vi "DigInputs Write.vi"(4 "error in (no error)":errorcluster, 5 "Value":string[](array[string]), 6 "Container State":T2, 7 "Display State In":T1) -> (0 "error out":errorcluster, 3 "Display State Out":T1)   [LabVIEW 2015, in "Input Criteria Table.xctl"]
uses:
  Input Criteria Table.xctl
  <vilib>/_xctls/Container State.ctl
  State.vi
  <vilib>/_xctls/XControlSupport.lvlib
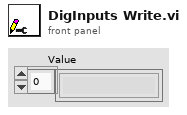
[diagram p1: front panel]
types:
  T1 = typedef "Input Criteria Table.xctl/State.vi" = cluster{"DI":string[], "Flags":string[]}
  T2 = typedef "XControlSupport.lvlib/Container State.ctl" = cluster{"Indicator?":bool, "Run Mode?":bool, " Refnum":refnum<vi>}
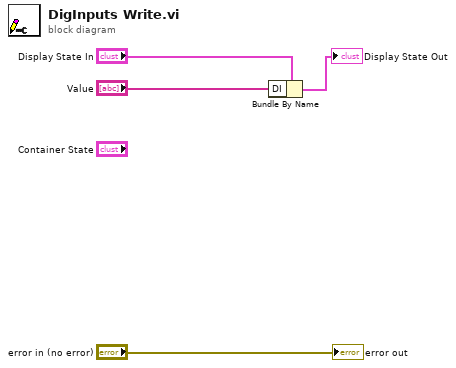
[diagram p0: block diagram]
diagram:
  n1 = Bundle By Name(cluster="Display State In", "DI"="Value") -> (→"Display State Out":T1)
  "error out" <- "error in (no error)"
